vi "RLS_Q5_block_Z.vi"(3 "P_k-1":dbl[][](array[numeric])=[[10000.0, 0.0, 0.0, 0.0, 0.0], [0.0, 10000.0, 0.0, 0.0, 0.0], [0.0, 0.0, 10000.0, 0.0, 0.0], [0.0, 0.0, 0.0, 10000.0, 0.0], [0.0, 0.0, 0.0, 0.0, 10000.0]], 4 "q_k-1":dbl[](array[numeric])=[1.0, 0.0, 0.0, 0.0, 0.0], 5 "ek":dbl format="%#_13g", 6 "phi":dbl[](array[numeric])=[0.0, 0.0, 0.0, 0.0, 0.0]) -> (0 "Pk":dbl[][](array[numeric]), 1 "qk":dbl[](array[numeric]), 2 "ek":dbl format="%#_13g")   [LabVIEW 2015]
panel:
  out "den":dbl
  out "num":dbl[](array[numeric])
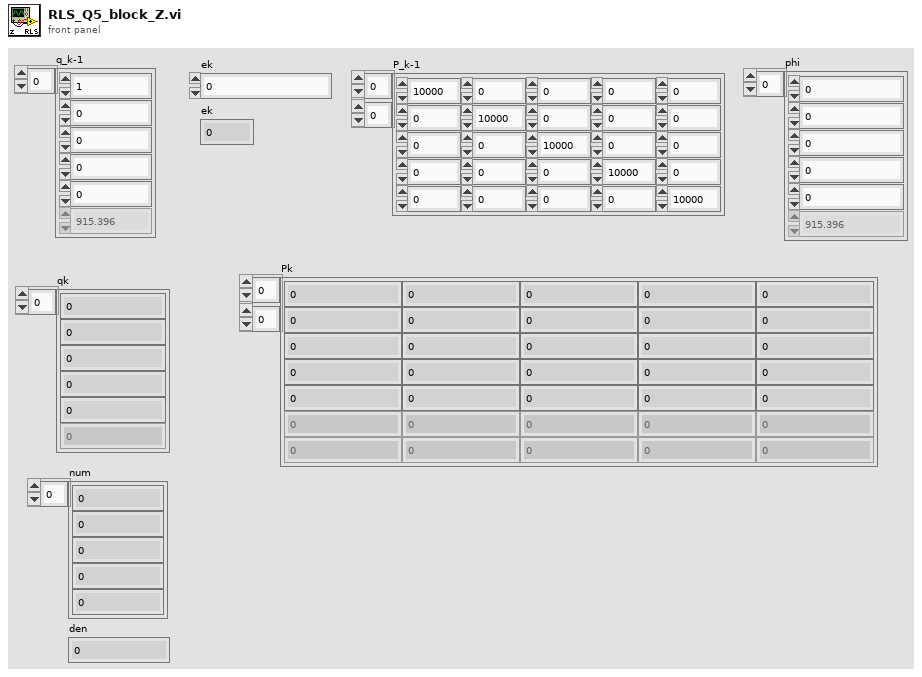
[diagram p1: front panel]
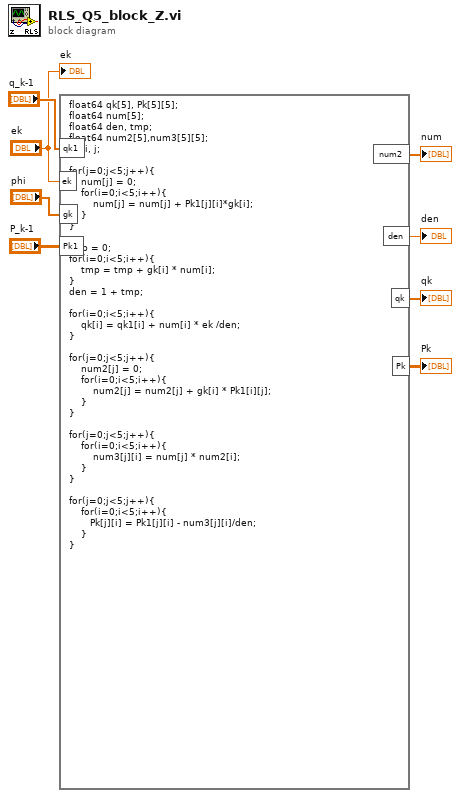
[diagram p0: block diagram]
diagram:
  n1 = formula code="float64 qk[5], Pk[5][5];\nfloat64 num[5];\nfloat64 den, tmp;\nfloat64 num2[5],num3[5][5];\nint i, j;\n\nfor(j=0;j<5;j++){\n    num[j] = 0;\n    for(i=0;i<5;i++){\n        num[j] = num[j] + Pk1[j][i]*gk[i];\n    }\n}\n\ntmp = 0;\nfor(i=0;i<5;i++){\n    tmp = tmp + gk[i] * num[i];\n}\nden = 1 + tmp;\n\nfor(i=0;i<5;i++){\n    qk[i] = qk1[i] + num[i] * ek /den;\n}\n\nfor(j=0;j<5;j++){\n    num2[j] = 0;\n    for(i=0;i<5;i++){\n        num2[j] = num2[j] + gk[i] * Pk1[i][j];\n    }\n}\n\nfor(j=0;j<5;j++){\n    for(i=0;i<5;i++){\n        num3[j][i] = num[j] * num2[i];\n    }\n}\n\nfor(j=0;j<5;j++){\n    for(i=0;i<5;i++){\n       Pk[j][i] = Pk1[j][i] - num3[j][i]/den;\n    }\n}"("ek"="ek", "qk1"="q_k-1", "Pk1"="P_k-1", "gk"="phi") -> ("num2"=→"num":dbl[], "den"=→"den":dbl, "qk"=→"qk":dbl[], "Pk"=→"Pk":dbl[][])
  "ek" <- "ek"
